vi "Create All Message Queues.vi"(8 "error in (no error)":errorcluster) -> (0 "error out":errorcluster, 3 "Message Queues out":T1)   [LabVIEW 2015, in "Message Queue.lvlib"]
doc: "This VI creates and initializes all the message queues for your application. If your application requires more than one message queue, right-click the \"Message Queues\" constant above and select Open Type Def. Add the new Message Queue(s) to the type definition, then initialize them in this VI."
uses:
  Message Queue.lvlib
  All Message Queues.ctl
  Message Cluster.ctl
  Enqueue Message (Single).vi
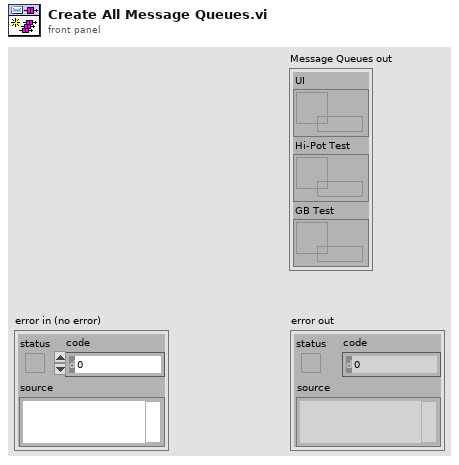
[diagram p1: front panel]
types:
  T1 = typedef "Message Queue.lvlib/All Message Queues.ctl" = cluster{"UI":refnum<queue>, "Hi-Pot Test":refnum<queue>, "GB Test":refnum<queue>}
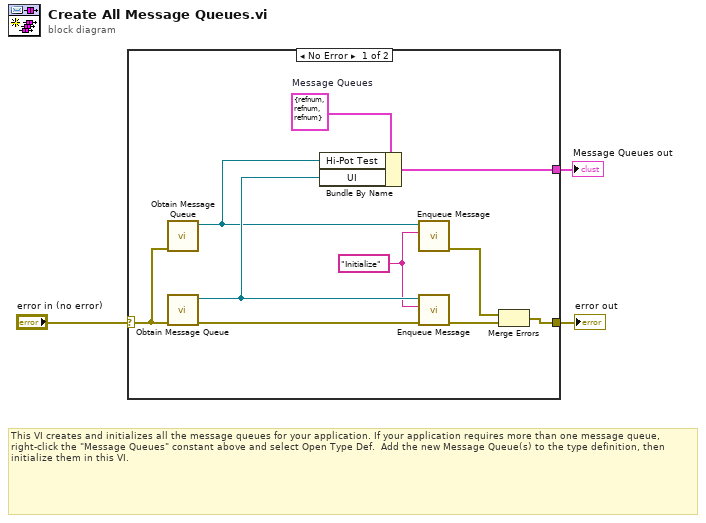
[diagram p0: block diagram]
diagram:
  # "This VI creates and initializes all the message queues for your application. If your application requires more than one message queue, right-click the \"Message Queues\" constant above and select Open Type Def.  Add the new Message Queue(s) to the type definition, then initialize them in this VI."
  n1 = case shown="No Error" "error in (no error)" {
    selector: "error in (no error)" -> [w8 w14]
    tunnel: [w5 w14] -> w3
    tunnel: [w11 _] -> w2
    frame No Error {
      w6 = "Initialize" ("Message")
      w12 = T1 {"UI"=refnum, "Hi-Pot Test"=refnum, "GB Test"=refnum}  # Message Queues
      n2 = call "Obtain Message Queue.vi"("error in (no error)"=w8) -> ("Message Queue"=w7:refnum<queue>)  [unwired: 9 in, 1 out]
      n3 = call "Obtain Message Queue.vi"("error in (no error)"=w8) -> ("error out"=w10:errorcluster, "Message Queue"=w9:refnum<queue>)  [unwired: 9 in]
      n4 = Bundle By Name(cluster=w12, "Hi-Pot Test"=w7, "UI"=w9) -> (w11:T1)
      n5 = call-poly "Enqueue Message.vi"("Message"=w6, "Message Queue"=w7) -> ("error out"=w4:errorcluster)  [unwired: 8 in, 1 out]
      n6 = call-poly "Enqueue Message.vi"("error in (no error)"=w10, "Message"=w6, "Message Queue"=w9) -> ("error out"=w13:errorcluster)  [unwired: 7 in, 1 out]
      n7 = Merge Errors(w4, w13) -> (w5:errorcluster)
    }
    frame Error {
    }
  }
  "Message Queues out" <- w2
  "error out" <- w3
